vi "Check Audio Device Already Configured.vi"(8 "error in (no error)":errorcluster, 11 "Audio Device Info":T1) -> (0 "error out":errorcluster, 3 "Device Configured":bool)   [LabVIEW 2020, in "G-Audio.lvlib"]
doc: "Check if an audio device has already been configured."
uses:
  G-Audio.lvlib
  Controls/Audio Device Info.ctl
  Controls/Audio Device Type.ctl
  Controls/Audio Device Format.ctl
  Controls/Audio Device Refnum.ctl
  Debug Path.vi
  Result To Error.vi
  MAX_DEVICES.vi
  <vilib>/Utility/file.llb/Application Directory.vi
  <vilib>/Utility/error.llb/Error Cluster From Error Code.vi
  Controls/Audio Device Native Data Format.ctl
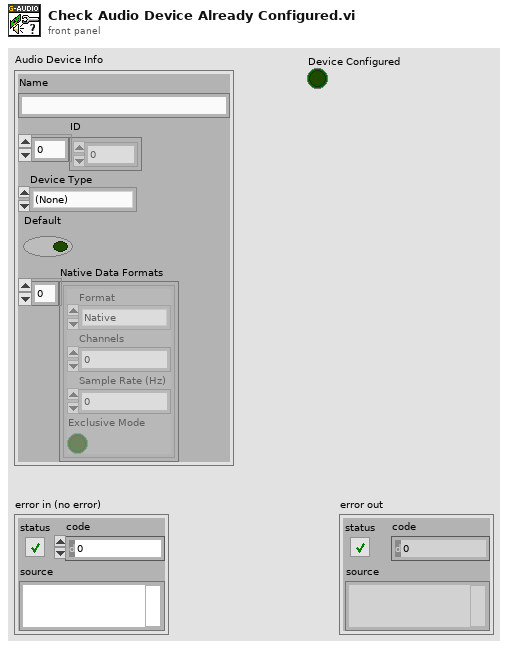
[diagram p1: front panel]
types:
  T1 = typedef "G-Audio.lvlib/Audio Device Info.ctl" = cluster{"Name":string, "ID":u8[], "Device Type":T2, "Default":bool, "Native Data Formats":T3[]}
  T2 = typedef "G-Audio.lvlib/Audio Device Type.ctl" = enum16{"(None)", "Playback", "Capture", "Duplex", "Loopback"}
  T3 = typedef "G-Audio.lvlib/Audio Device Native Data Format.ctl" = cluster{"Format":T4, "Channels":u32, "Sample Rate (Hz)":u32, "Exclusive Mode":bool}
  T4 = typedef "G-Audio.lvlib/Audio Device Format.ctl" = enum16{"Native", "U8", "I16", "I32", "SGL"}
  T5 = typedef "G-Audio.lvlib/Audio Device Refnum.ctl" = refnum<file>
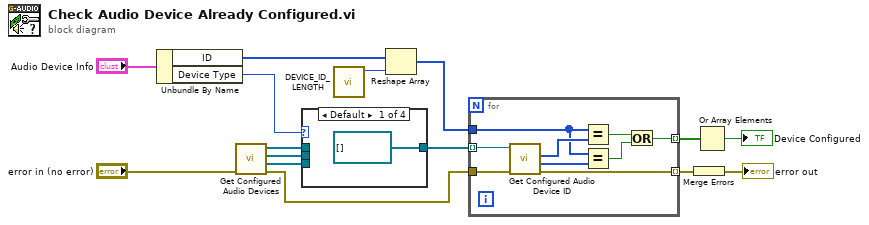
[diagram p0: block diagram]
diagram:
  n1 = Unbundle By Name("Audio Device Info") -> ("ID"=w9:u8[], "Device Type"=w4:T2)
  n2 = call "Get Configured Audio Devices.vi"("error in (no error)"="error in (no error)") -> ("error out"=w3:errorcluster, "Loopback Device Refnums"=w12:T5[], "Capture Device Refnums"=w13:T5[], "Playback Device Refnums"=w14:T5[])  [unwired: 7 in]
  n3 = case shown="Default" w4 {
    tunnel: w14 -> [_ w17 _ _]
    tunnel: w13 -> [_ _ w18 _]
    tunnel: w12 -> [_ _ _ w19]
    tunnel: [T5[] [] ("Loopback Device Refnums") w17 w18 w19] -> w11
    frame Default {
    }
    frame "Playback" {
    }
    frame "Capture" {
    }
    frame "Loopback" {
    }
  }
  n4 = call "DEVICE_ID_LENGTH.vi"() -> ("DEVICE_ID_LENGTH"=w10:i32)  [unwired: 11 in]
  n5 = Reshape Array(w9, w10) -> (w8:u8[])
  n6 = for {
    tunnel: w11 -> [w28] mode=indexing
    tunnel: w8 -> [w20]
    tunnel: [w23] -> w7 mode=indexing
    tunnel: w3 -> [w22]
    tunnel: [w21] -> w2 mode=indexing
    n7 = call "Get Configured Audio Device ID.vi"("error in (no error)"=w22, "Audio Device Refnum In"=w28) -> ("error out"=w21:errorcluster, "Actual Device ID"=w26:u8[], "Configured Device ID"=w27:u8[])  [unwired: 6 in, 1 out]
    n8 = Equal?(x=w20, y=w27) -> (x = y?=w25:bool)
    n9 = Equal?(x=w20, y=w26) -> (x = y?=w24:bool)
    n10 = Or(x=w25, y=w24) -> (x .or. y?=w23:bool)
  }
  n11 = Merge Errors(w2) -> (→"error out":errorcluster)
  n12 = Or Array Elements(Boolean array=w7) -> (logical OR=→"Device Configured":bool)
